vi "sequencerTopLevel.vi"() -> ()   [LabVIEW 2014]
uses:
  sequencerState.ctl
  <vilib>/rvi/Emulation/niFpgaGetClockAttributes.vi
  <vilib>/rvi/Emulation/niFpgaSctlEmulationGetInTimedLoop.vi
  <vilib>/rvi/Emulation/niFpgaEmulationReportErrorSimple.vi
  <vilib>/rvi/Emulation/niFpgaProcessEmulError.vi
  <vilib>/rvi/interface/RandomDataEmulation/niFpgaRandomDataHandleErrors.vi
  <vilib>/rvi/Emulation/niFpgaCriticalErrorInLSC.vi
  <vilib>/rvi/DataTransferAndStorage/Container/XNode/niFpgaContainer.xnode
  <vilib>/rvi/interface/RandomDataEmulation/nirviRandomDataFpgaReadWriteTemplate.vi
panel:
  in  "nOfScanRegions":i32
  in  "Reset":bool
  in  "waitForKepco /t":u32=2000
  in  "Halt":bool
  in  "nOfCycles":i32 format="%0d"
  in  "nOfLoops":i32 format="%0d"
  out "timeOutSetVolt":bool
  out "Scanning":bool=TRUE
  in  "Abort":bool
  in  "start":bool
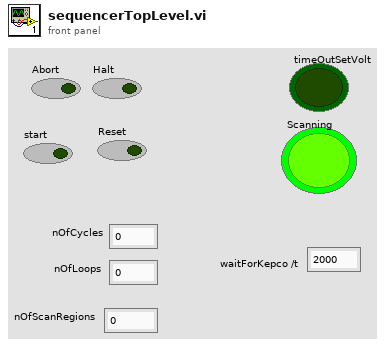
[diagram p1: front panel]
types:
  T1 = typedef "sequencerState.ctl" = enum16{"init", "idle", "readTracks", "scan"}
  T2 = cluster{"SCLK":refnum<k21>, "CS":refnum<k21>, "MOSI":refnum<k21>, "MISO":refnum<k21>}
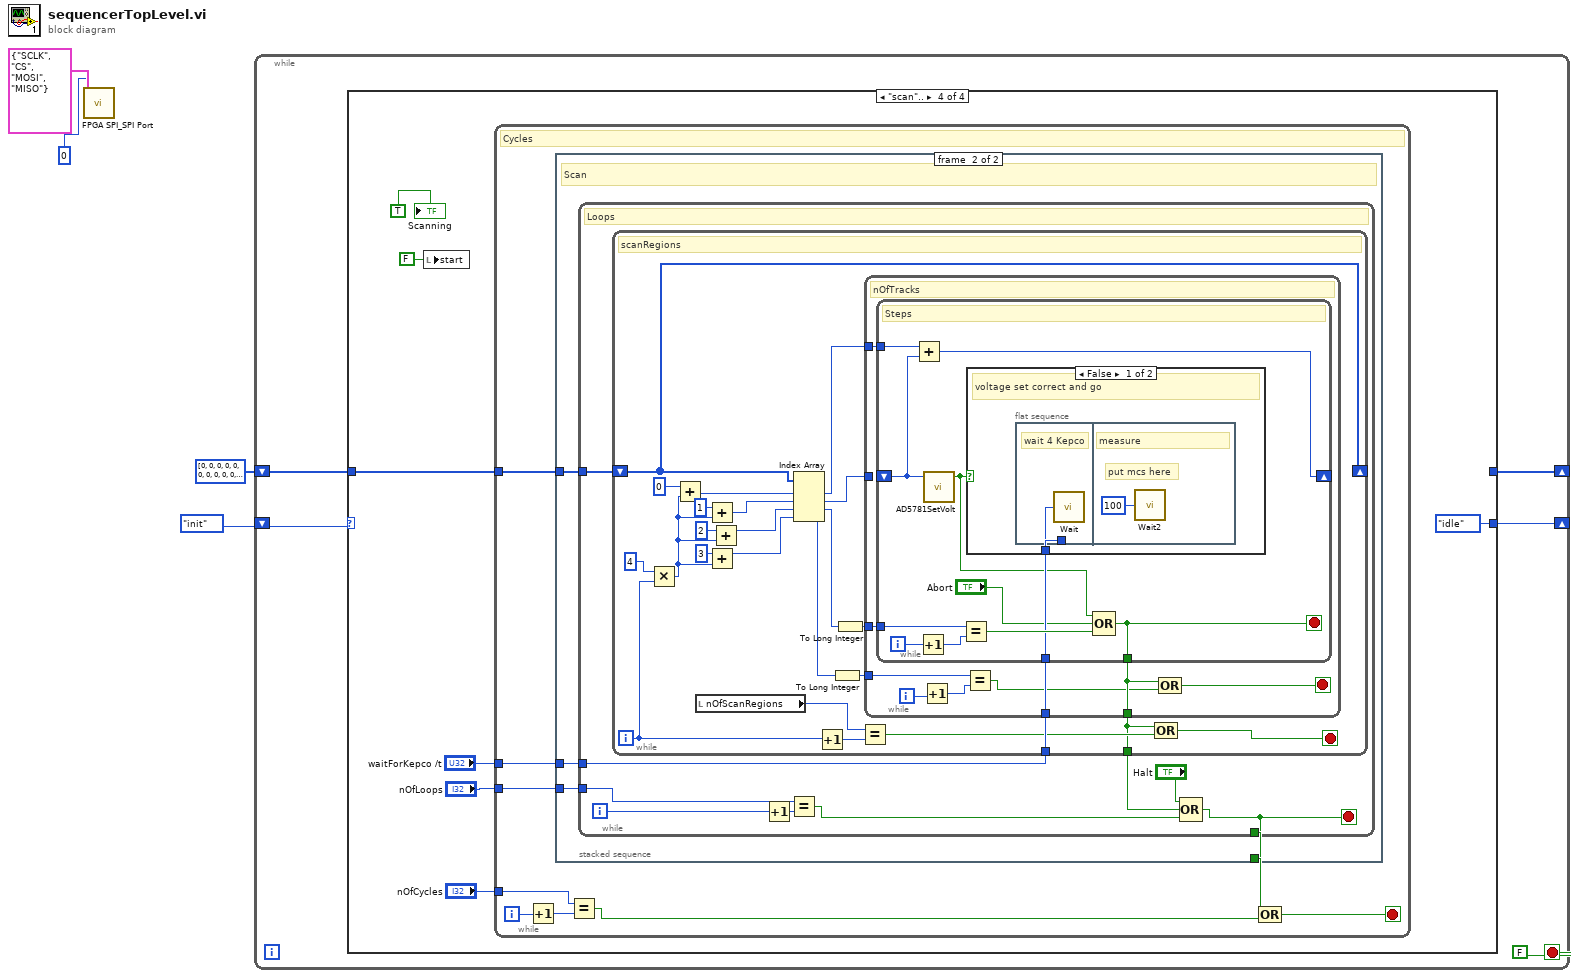
[diagram p0: block diagram]
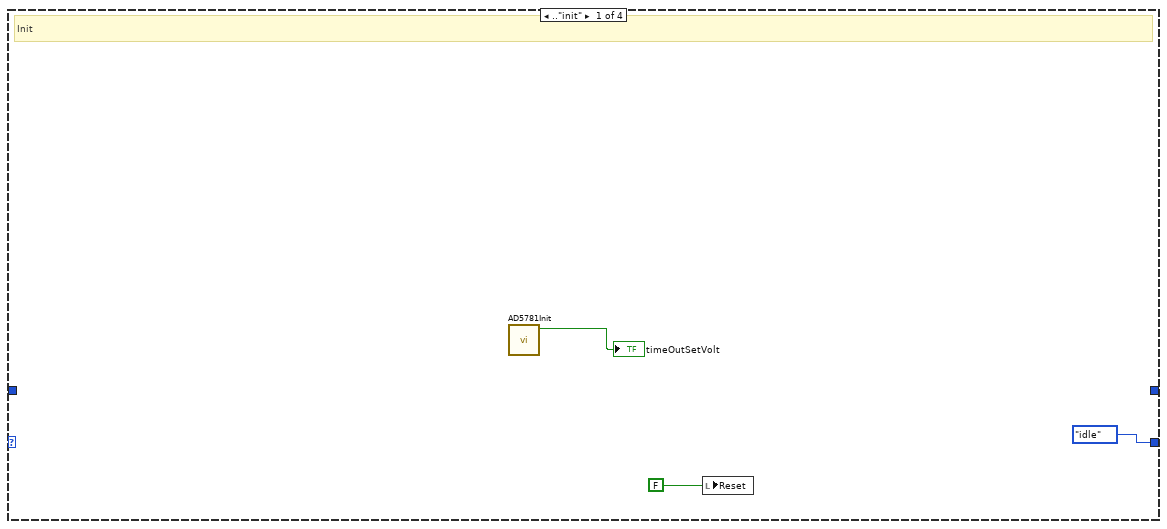
[diagram p2: hidden frame]
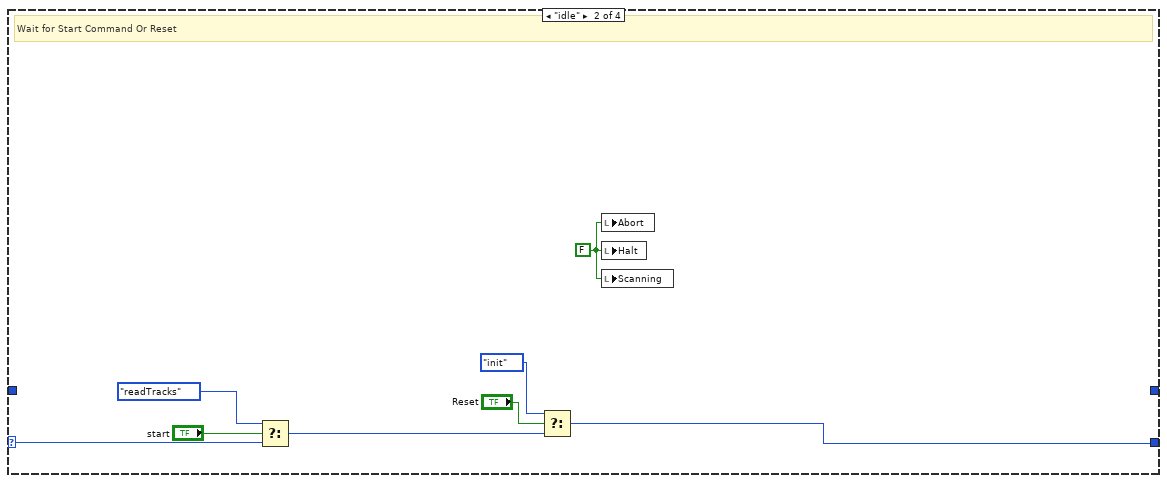
[diagram p3: hidden frame]
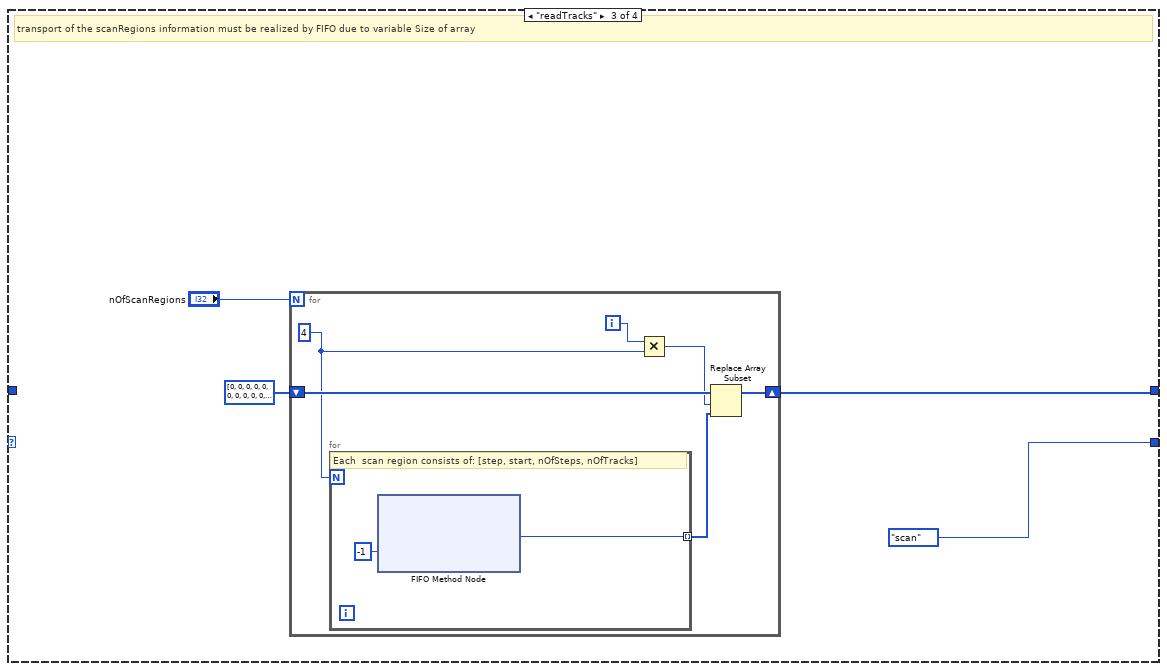
[diagram p4: hidden frame]
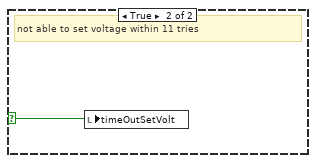
[diagram p6: hidden frame]
diagram:
  n1 = call "FPGA SPI_SPI Port.vi"("Port"=i8 0, "FPGA IO"=T2 {"SCLK"="SCLK", "CS"="CS", "MOSI"="MOSI", "MISO"="MISO"}) -> ()  [unwired: 10 in]
  n2 = while {
    shift-right: [w8] -> _
    shift-left: sequencerState."init" ("Enum") -> [w9]
    shift-right: [w6] -> _
    shift-left: u32[] [0, 0, 0, 0, 0, 0, 0, 0, 0, 0, 0, 0, 0, 0, 0, 0, 0, 0, 0, 0, 0, 0, 0, 0, 0, 0, 0, 0, 0, 0, 0, 0, 0, 0, 0, 0, 0, 0, 0, 0, 0, 0, 0, 0, 0, 0, 0, 0, 0, 0, 0, 0, 0, 0, 0, 0, 0, 0, 0, 0, 0, 0, 0, 0, 0, 0, 0, 0, 0] -> [w5]
    stop <- FALSE stop-if-true
    n3 = case shown="\"scan\".." w9 {
      selector: w9 -> [_ w20 _ _]
      tunnel: [sequencerState."idle" ("Enum") w16 sequencerState."scan" ("Enum") sequencerState."idle" ("Enum")] -> w8
      tunnel: [_ _ w22 _] -> w6
      tunnel: w5 -> [_ _ _ w33]
      frame .."init" {
        # "Init"
        n4 = call "AD5781Init.vi"() -> ("timeOut"=→"timeOutSetVolt":bool)  [unwired: 11 in]
        n5 = local write "Reset"(FALSE ("Reset")) -> ()
      }
      frame "idle" {
        w13 = FALSE ("Abort")
        # "Wait for Start Command Or Reset"
        n6 = Select(t=sequencerState."readTracks", s="start", f=w20) -> (s? t:f=w17:T1)
        n7 = Select(t=sequencerState."init", s="Reset", f=w17) -> (s? t:f=w16:T1)
        n8 = local write "Abort"(w13) -> ()
        n9 = local write "Halt"(w13) -> ()
        n10 = local write "Scanning"(w13) -> ()
      }
      frame "readTracks" {
        # "transport of the scanRegions information must be realized by FIFO due to variable Size of array"
        n11 = for {
          N: "nOfScanRegions" -> [_]
          shift-right: [w29] -> w22
          shift-left: u32[] [0, 0, 0, 0, 0, 0, 0, 0, 0, 0, 0, 0, 0, 0, 0, 0, 0, 0, 0, 0, 0, 0, 0, 0, 0, 0, 0, 0, 0, 0, 0, 0, 0, 0, 0, 0, 0, 0, 0, 0, 0, 0, 0, 0, 0, 0, 0, 0, 0, 0, 0, 0, 0, 0, 0, 0, 0, 0, 0, 0, 0, 0, 0, 0, 0, 0, 0, 0, 0] -> [w30]
          i -> [w27]
          w26 = 4 ("y")
          n12 = for {
            N: w26 -> [_]
            tunnel: [w32] -> w28 mode=indexing
            # "Each  scan region consists of: [step, start, nOfSteps, nOfTracks]"
            n13 = xnode ("FIFO Method Node")("Timeout"=-1) -> ("Element"=w32:u32)  [unwired: 1 in, 2 out]
          }
          n14 = Multiply(x=w27, y=w26) -> (x*y=w25:i32)
          n15 = Replace Array Subset(array=w30, new element=w28, index=w25) -> (w29:u32[])
        }
      }
      frame "scan".. {
        n16 = local write "start"(FALSE ("start")) -> ()
        n17 = while {
          tunnel: "nOfLoops" -> [w48]
          tunnel: "nOfCycles" -> [w45]
          tunnel: "waitForKepco /t" -> [w41]
          tunnel: w33 -> [w40]
          i -> [w47]
          stop <- w43 stop-if-true
          # "Cycles"
          n18 = Increment(x=w47) -> (x+1=w46:i32)
          n19 = stacked-sequence {
            tunnel: w48 -> [_ w52]
            tunnel: [_ w51] -> w42
            tunnel: w41 -> [_ w50]
            tunnel: w40 -> [_ w49]
            frame #0 {
              # "HOW to communicate with Agilent/DMM?"
              # "Measure Voltage"
            }
            frame #1 {
              # "Scan"
              n20 = while {
                tunnel: w52 -> [w60]
                tunnel: [w56] -> w51
                tunnel: w50 -> [w55]
                tunnel: w49 -> [w53]
                i -> [w61]
                stop <- w56 stop-if-true
                # "Loops"
                n21 = while {
                  tunnel: [w74] -> w57
                  tunnel: w55 -> [w85]
                  shift-right: [w72] -> _
                  shift-left: w53 -> [w72]
                  i -> [w68]
                  stop <- w77 stop-if-true
                  # "scanRegions"
                  n22 = Multiply(x=4 ("y"), y=w68) -> (x*y=w62:i32)
                  n23 = Add(x=0 ("index"), y=w62) -> (x+y=w67:i32)
                  n24 = local read "nOfScanRegions"() -> (w73:i32)
                  n25 = Add(x=1 ("index"), y=w62) -> (x+y=w65:i32)
                  n26 = Add(x=3 ("index"), y=w62) -> (x+y=w63:i32)
                  n27 = Add(x=2 ("index"), y=w62) -> (x+y=w64:i32)
                  n28 = Index Array(array=w72, index #1=w67, index #2=w65, index #3=w64, index #4=w63) -> (element #1=w81:u32, element #2=w80:u32, element #3=w71:u32, element #4=w70:u32)
                  n29 = Increment(x=w68) -> (x+1=w76:i32)
                  n30 = To Long Integer(number=w70) -> (32bit integer=w78:i32)
                  n31 = To Long Integer(number=w71) -> (32bit integer=w79:i32)
                  n32 = Equal?(x=w73, y=w76) -> (x = y?=w75:bool)
                  n33 = while {
                    tunnel: [w91] -> w74
                    tunnel: w85 -> [w92]
                    tunnel: w81 -> [w88]
                    tunnel: w80 -> [_]
                    tunnel: w79 -> [w87]
                    tunnel: w78 -> [w86]
                    i -> [w93]
                    stop <- w89 stop-if-true
                    # "nOfTracks"
                    n34 = while {
                      shift-right: [w103] -> _
                      shift-left: _ -> [w100]
                      tunnel: [w101] -> w91
                      tunnel: w92 -> [w99]
                      tunnel: w88 -> [w95]
                      tunnel: w87 -> [w96]
                      i -> [w105]
                      stop <- w101 stop-if-true
                      # "Steps"
                      n35 = Add(x=w95, y=w100) -> (x+y=w103:u32)
                      n36 = Increment(x=w105) -> (x+1=w102:i32)
                      n37 = call "AD5781SetVolt.vi"("SetVolt"=w100) -> ("timedOut"=w97:bool)  [unwired: 4 in]
                      n38 = Equal?(x=w96, y=w102) -> (x = y?=w104:bool)
                      n39 = case shown="False" w97 {
                        selector: w97 -> [_ w109]
                        tunnel: w99 -> [w106 _]
                        frame False {
                          # "voltage set correct and go"
                          n40 = flat-sequence {
                            tunnel: w106 -> [w107]
                            frame #0 {
                              # "wait 4 Kepco"
                              n41 = call "Wait"("Count(Ticks)"=w107) -> ()  [unwired: 1 out]
                            }
                            frame #1 {
                              # "put mcs here"
                              # "measure"
                              n42 = call "Wait2"("Count(mSec)"=u8 100) -> ()  [unwired: 1 out]
                            }
                          }
                        }
                        frame True {
                          # "not able to set voltage within 11 tries"
                          n43 = local write "timeOutSetVolt"(w109) -> ()
                        }
                      }
                      n44 = Compound Arithmetic op=OR(w97, "Abort", w104) -> (w101:bool)
                    }
                    n45 = Increment(x=w93) -> (x+1=w94:i32)
                    n46 = Equal?(x=w86, y=w94) -> (x = y?=w90:bool)
                    n47 = Compound Arithmetic op=OR(w91, w90) -> (w89:bool)
                  }
                  n48 = Compound Arithmetic op=OR(w74, w75) -> (w77:bool)
                }
                n49 = Increment(x=w61) -> (x+1=w58:i32)
                n50 = Equal?(x=w60, y=w58) -> (x = y?=w59:bool)
                n51 = Compound Arithmetic op=OR("Halt", w57, w59) -> (w56:bool)
              }
            }
          }
          n52 = Equal?(x=w45, y=w46) -> (x = y?=w44:bool)
          n53 = Compound Arithmetic op=OR(w42, w44) -> (w43:bool)
        }
        "Scanning" <- TRUE
      }
    }
  }
